vi "UpdateStimQueueStimulus.vi"(8 "error in (no error)":errorcluster, 11 "Stimulus in":refnum<class "Stimulus.lvclass">) -> (0 "error out":errorcluster, 3 "Stimulus out":refnum<class "Stimulus.lvclass">)   [LabVIEW 2014, in "Stimulus.lvclass"]
uses:
  Stimulus.lvclass
  Stimulus.lvclass/Stimulus.ctl
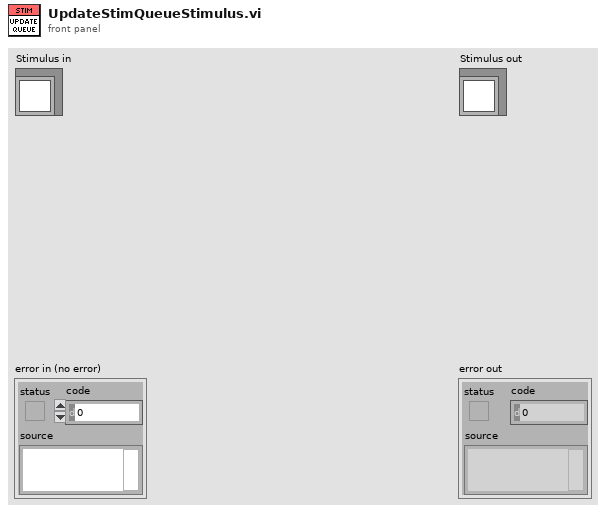
[diagram p1: front panel]
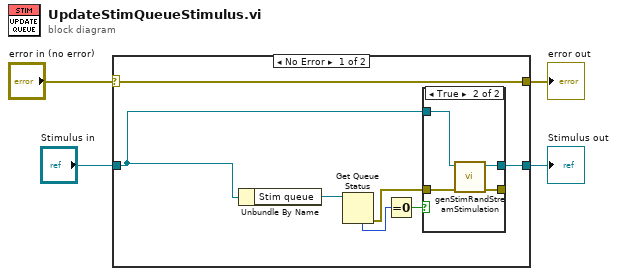
[diagram p0: block diagram]
diagram:
  n1 = case shown="No Error" "error in (no error)" {
    selector: "error in (no error)" -> [w11 w19]
    tunnel: [w11 w19] -> w3
    tunnel: [w6 w18] -> w1
    tunnel: "Stimulus in" -> [w5 w18]
    frame No Error {
      n2 = Unbundle By Name(w5) -> ("Stim queue"=w7:refnum<queue>)
      n3 = Get Queue Status(queue=w7) -> (error out=w10:errorcluster, # elements in queue=w8:i32)  [unwired: 2 in, 6 out]
      n4 = Equal To 0?(x=w8) -> (x = 0?=w9:bool)
      n5 = case shown="True" w9 {
        tunnel: [w13 w16] -> _
        tunnel: w10 -> [w13 w17]
        tunnel: w5 -> [w12 w15]
        tunnel: [w12 w14] -> w6
        frame False {
        }
        frame True {
          n6 = call-dynamic "genStimRandStreamStimulation.vi"("error in (no error)"=w17, "Stimulus in"=w15) -> ("error out"=w16:errorcluster, "Stimulus out"=w14:refnum<class "Stimulus.lvclass">)  [unwired: 8 in]
        }
      }
    }
    frame Error {
    }
  }
  "error out" <- w3
  "Stimulus out" <- w1
